vi "Main.vi"() -> ()   [LabVIEW 2019]
doc: "The myRIO Project template acquires acceleration data from the onboard accelerometer and displays the changes of acceleration values in a waveform chart."
uses:
  <vilib>/myRIO/Common/Instrument Driver Framework/myRIO v1.0/Encoder/typedefs/Encoder Signal Mode.ctl
  <vilib>/myRIO/Instrument Drivers/Onboard IO/Encoder/typedefs/Encoder Reference.ctl
  <vilib>/myRIO/Common/Instrument Driver Framework/Utilities/typedefs/myRIO Generic Hardware Reference.ctl
  <vilib>/myRIO/Common/Instrument Driver Framework/Utilities/typedefs/Hardware Version Enum.ctl
  <vilib>/myRIO/Common/Instrument Driver Framework/Utilities/typedefs/myRIO v1.0 Reference.ctl
  <vilib>/myRIO/Common/Instrument Driver Framework/Utilities/typedefs/Generic FPGA Reference.ctl
  <vilib>/myRIO/Common/Instrument Driver Framework/myRIO v1.0/Encoder/typedefs/Encoder Channels Enum.ctl
  <vilib>/myRIO/Common/Instrument Driver Framework/myRIO v1.0/Encoder/typedefs/Encoder Configuration v1.0.ctl
  <vilib>/userDefined/High Color/nirio_resource_hc.ctl
  <vilib>/Simulation/Scripting/Companion Diagram/SimConfigNode/SimParams.ctl
  <vilib>/Simulation/Scripting/Companion Diagram/SimConfigNode/_simSolvers.ctl
  <vilib>/Simulation/Implementation/Shared/SIMSCR Execution Mode.ctl
  <vilib>/Simulation/Param Hierarchy/Typedefs/SIMPH Param Control Actions.ctl
  <vilib>/myRIO/Common/Instrument Driver Framework/Utilities/vis/Is FPGA Ref Available.vi
  <vilib>/myRIO/Common/Instrument Driver Framework/myRIO v1.0/Encoder/vis/myRIO v1.1 Open Encoder.vi
  <vilib>/myRIO/Instrument Drivers/Onboard IO/Encoder/vis/Read.vi
  <vilib>/Simulation/Implementation/Shared/NILVSim_ParamChanged.vi
  <vilib>/Simulation/Implementation/Shared/NILVSIM_BeginStep.vi
  <vilib>/Simulation/Implementation/Shared/NILVSim_Manager.vi
  <vilib>/Utility/error.llb/Clear Errors.vi
  <vilib>/Simulation/Implementation/Shared/NILVSim_FinalizeModel.vi
  <vilib>/myRIO/Common/Instrument Driver Framework/Utilities/vis/Validate Channels.vi
  <vilib>/myRIO/Common/Instrument Driver Framework/myRIO v1.0/Encoder/vis/myRIO v1.0 Reserve Encoder.vi
  <vilib>/myRIO/Common/Instrument Driver Framework/myRIO v1.0/UART/vis/myRIO v1.0 Close UART.vi
  <vilib>/myRIO/Common/Instrument Driver Framework/myRIO v1.0/Encoder/vis/myRIO v1.0 Build MUX Configuration Encoder.vi
  <vilib>/myRIO/Common/Instrument Driver Framework/myRIO v1.0/Resource Manager/vis/myRIO v1.0 Reserve Channel List.vi
  <vilib>/myRIO/Common/Instrument Driver Framework/myRIO v1.0/Resource Manager/vis/myRIO v1.0 Create Configuration List.vi
  <vilib>/myRIO/Common/Instrument Driver Framework/myRIO v1.0/Resource Manager/vis/myRIO v1.0 Reserve Channel.vi
  <vilib>/myRIO/Common/Instrument Driver Framework/myRIO v1.0/Resource Manager/vis/myRIO v1.0 Unreserve Channel.vi
  <vilib>/myRIO/Common/Instrument Driver Framework/myRIO v1.0/Resource Manager/vis/myRIO v1.0 Build Mutex Name.vi
  <vilib>/Utility/VariantDataType/GetNumericInfo.vi
  <vilib>/Utility/error.llb/Error Cluster From Error Code.vi
  <vilib>/myRIO/Common/Instrument Driver Framework/myRIO v1.0/myRIO v1.1 Open.vi
  <vilib>/myRIO/Common/Instrument Driver Framework/Utilities/vis/IO Manager.vi
  <vilib>/myRIO/Common/Instrument Driver Framework/Utilities/vis/Configuration Manager.vi
  <vilib>/myRIO/Common/Instrument Driver Framework/myRIO v1.0/Resource Manager/vis/myRIO v1.0 Configure IO.vi
  <vilib>/myRIO/Common/Instrument Driver Framework/myRIO v1.0/myRIO v1.0 Close.vi
  <vilib>/myRIO/Common/Instrument Driver Framework/myRIO v1.0/Encoder/vis/myRIO v1.0 Configure Encoder.vi
  <vilib>/myRIO/Common/Instrument Driver Framework/myRIO v1.0/Encoder/vis/myRIO v1.0 Read Encoder.vi
  <vilib>/Simulation/Implementation/Shared/SIM Unbundle Sim Info.vi
  <vilib>/Simulation/Implementation/Shared/NILVSim_Initialize.vi
  <vilib>/Simulation/Utility/Implementation/NILVSim Get Time and IsAcceptedStep.vi
  <vilib>/Simulation/Implementation/Shared/SIMSH Read Queue.vi
  <vilib>/Simulation/Implementation/Shared/NILVSim_GetModelError.vi
  <vilib>/Simulation/Implementation/Shared/SIM Bundle Sim Info.vi
  <vilib>/Utility/file.llb/Write Delimited Spreadsheet (DBL).vi
  <vilib>/myRIO/Common/Instrument Driver Framework/Utilities/vis/FPGA Ref Manager.vi
  <vilib>/myRIO/Common/Instrument Driver Framework/myRIO v1.0/myRIO v1.0 Reset FPGA.vi
  <vilib>/myRIO/Common/Instrument Driver Framework/myRIO v1.0/IRQ/vis/myRIO v1.0 IRQ Info FGV.vi
  <vilib>/myRIO/Common/Instrument Driver Framework/myRIO v1.0/IRQ/vis/myRIO v1.0 Timer IRQ Info FGV.vi
  <vilib>/myRIO/Common/Instrument Driver Framework/myRIO v1.0/IRQ/vis/myRIO v1.0 ISR Agent.vi
  <vilib>/myRIO/Instrument Drivers/Utilities/vis/Reset Index.vi
  <vilib>/myRIO/Common/Instrument Driver Framework/myRIO v1.0/Resource Manager/vis/myRIO v1.0 Block Write Resource Manager.vi
  <vilib>/myRIO/Express VI/Onboard IO/Encoder/Encoder Express VI.xnode
  <vilib>/myRIO/Common/Instrument Driver Framework/myRIO v1.0/Encoder/typedefs/Encoder Count Direction Enum.ctl
  <vilib>/myRIO/Instrument Drivers/Onboard IO/Encoder/vis/myRIO Encoder Open.xnode
  <vilib>/Simulation/Implementation/XNodeFramework/SimXNode/SimX.xnode
  Sub_OBS.vi
  <vilib>/Simulation/Scripting/Companion Diagram/SimConfigNode/SimDog.xnode
  <vilib>/myRIO/Instrument Drivers/Onboard IO/Encoder/Encoder.lvlib
  <vilib>/myRIO/Instrument Drivers/Utilities/Utilities.lvlib
  <vilib>/Simulation/Implementation/Shared/NI_SIM_Implementation.lvlib
panel:
  out "error out":errorcluster
  in  "Stop 2":bool
  out "Direction 1":enum16{"Counting Up", "Counting Down"}(ring)
  out "Overflow? 1":bool
  in  "Reset":bool
  out "Graph 3":T1(graph)
  in  "Freq[Hz]":dbl=1000.0
  out "Direction 2":enum16{"Counting Up", "Counting Down"}(ring)
  out "Overflow? 2":bool
  in  "Reset 2":bool
  out "ref pos 2":dbl
  out "Duty Cycle out 2":dbl=0.5
  out "Duty Cycle out":dbl=0.5
  in  "k_OBS":dbl
  in  "b_OBS":dbl=1.0
  in  "b_TAR":dbl
  in  "k_TAR":dbl=1.0
  out "Graph 2":cluster{dbl, "x2hat":dbl}(graph)
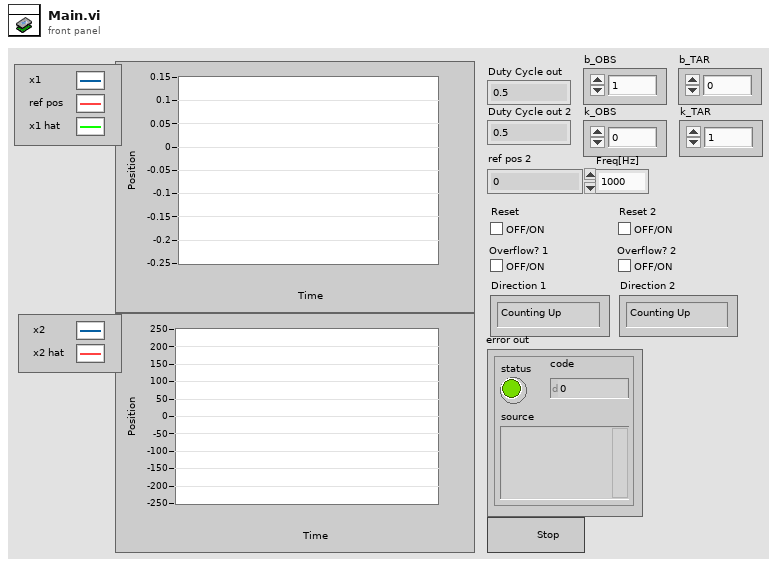
[diagram p1: front panel]
types:
  T1 = cluster{"ave out":dbl, "ave out":dbl, "x1hat":dbl}
  T2 = enum16{"Simulate to Completion", "Single Time-Step Simulation (Fixed Step Only)"}
  T3 = typedef "SIMSCR Execution Mode.ctl" = enum16{"Simulate to Completion", "Single Time-Step Simulation (Fixed Step Only)"}
  T4 = typedef "SIMPH Param Control Actions.ctl" = enum16{"get params", "set params"}
  T5 = cluster{"SIMSH Sim Time":dbl, "Sum 3":cluster{"Result":dbl}, "L2":cluster{"output":dbl}, "L1":cluster{"output":dbl}, "Summation 2":cluster{"Result":dbl}, "Formula Node":cluster{"AI":dbl, "BI":dbl, "L1":dbl, "L2":dbl}, "A/I":cluster{"output":dbl}, "2":cluster{"output":dbl}, "1":cluster{"output":dbl}, "Summation":cluster{"Result":dbl}, "B/I":cluster{"output":dbl}}
  T6 = typedef "SimParams.ctl" = cluster{"Initial Time (s)":dbl, "Final Time (s)":dbl, "Step Size (s)":dbl, "ODE Solver":T7, "Minimum Step Size (s)":dbl, "Maximum Step Size (s)":dbl, "Relative Tolerance":dbl, "Absolute Tolerance":dbl, "Software Timing":bool, "Initial Step Size (s)":dbl, "Automatic Fixed Step Size?":bool, "Automatic Discrete Step Size?":bool, "Discrete Step Size (s)":dbl, "Calculate using Time Step":bool, "Solver Wired?":bool, "Prev.Frm.Expected End":u64, "Prev.Frm.Actual End":u64, "Prev.Frm.Finished Late?":bool, "Prev.Iter.Expected End":u64, "Prev.Iter.Actual End":u64, "Prev.Iter.Finished Late?":bool, "Expected Iteration Start":u64, "Actual Iteration Start":u64, "Expected Frame Start":u64, "Actual Frame Start":u64, "Source Name":string, "Name":string, "Period":i64, "Deadline":i64, "Offset":i64, "Start":i64, "Priority":i32, "Timeout":i32, "Processor":i32, "Mode":enum32{"No Change", "Process missed periods, maintain original phase", "Discard missed periods, maintain original phase", "Process missed periods, ignore original phase", "Discard missed periods, ignore original phase"}, "Wakeup reason":enum32{"Normal", "Aborted", "Asynchronous wakeup", "Timing source error", "Timed loop error", "Timeout"}, "Error":errorcluster, "Source Type":string, "Secondary Source Type":string, "Global End Time":u64, "Global Start Time":u64, "Full Solver Reset":bool, "Execution Mode":T3, "Nan/Inf Check":bool, "Custom Solver Library":string, "Solver Is Variable":bool, "custom solver name":string, "Signal Collection Decimation":u32}
  T7 = typedef "_simSolvers.ctl" = enum16{"Runge-Kutta 1 (Euler)", "Runge-Kutta 2", "Runge-Kutta 3", "Runge-Kutta 4", "Runge-Kutta 23 (variable)", "Runge-Kutta 45 (variable)", "BDF (variable)", "Adams-Moulton (variable)", "Rosenbrock (variable)", "Discrete States Only", "SDIRK 4 (variable)", "Radau 5 (variable)", "Radau 9 (variable)", "Radau 13 (variable)", "Radau [Variable Order] (variable)", "Gear's Method (variable)", "Linearizer", "State Query", "Trim Eval", "Custom Solver"}
  T8 = typedef "Encoder.lvlib/Encoder Reference.ctl" = cluster{"myRIO Reference":T9, "Encoder Channels Enum":T13}
  T9 = typedef "myRIO Generic Hardware Reference.ctl" = cluster{"myRIO Model":T10, "myRIO Hardware Reference":T11}
  T10 = typedef "Hardware Version Enum.ctl" = enum16{"Unknown", "myRIO-1900", "myRIO-1950", "roboRIO", "NI ELVIS RIO CM", "ELVIS III"}
  T11 = typedef "myRIO v1.0 Reference.ctl" = cluster{"Generic FPGA Reference":T12, "Allow multiple opens":bool}
  T12 = typedef "Generic FPGA Reference.ctl" = refnum<k20>
  T13 = typedef "Encoder Channels Enum.ctl" = enum16{"Not Connected", "C/ENC0", "C/ENC1", "A/ENC", "A/ENC0", "A/ENC1", "A/ENC2", "A/ENC3", "A/ENC4", "A/ENC5", "A/ENC6", "A/ENC7", "A/ENC8", "A/ENC9", "B/ENC", "B/ENC0", "B/ENC1", "B/ENC2", "B/ENC3", "B/ENC4", "B/ENC5", "B/ENC6", "B/ENC7", "B/ENC8", "B/ENC9", "DIO/ENC0", "DIO/ENC1", "DIO/ENC2", "DIO/ENC3", "DIO/ENC4"}
  T14 = typedef "Encoder Signal Mode.ctl" = enum16{"Quadrature phase signal", "Step and direction signal"}
  T15 = typedef "nirio_resource_hc.ctl" = tag
  T16 = typedef "Encoder Count Direction Enum.ctl" = enum16{"Counting Up", "Counting Down"}
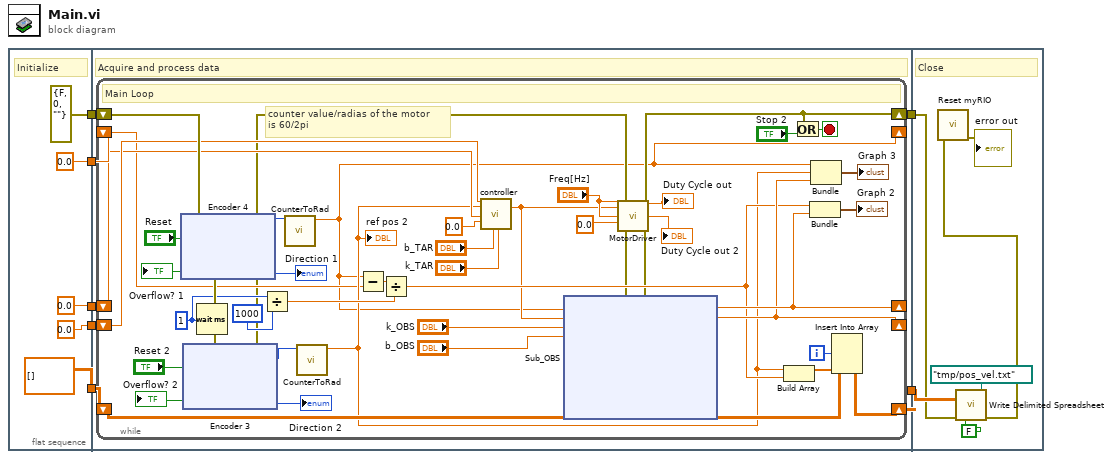
[diagram p0: block diagram]
diagram:
  n1 = flat-sequence {
    tunnel: [errorcluster {"status"=FALSE, "code"=0, "source"=""} ("error in (no error)")] -> w7
    tunnel: [dbl[][] [] ("array")] -> w6
    tunnel: [0.0 ("rads")] -> w5
    tunnel: [0.0 ("rads")] -> w4
    tunnel: [0.0 ("rads")] -> w3
    tunnel: w7 -> [w19]
    tunnel: w6 -> [w18]
    tunnel: [w17] -> w2
    tunnel: [w16] -> w1
    tunnel: w5 -> [w15]
    tunnel: w4 -> [w14]
    tunnel: w3 -> [w13]
    tunnel: w2 -> [w430]
    tunnel: w1 -> [w431]
    frame #0 {
      # "Initialize"
    }
    frame #1 {
      # "Acquire and process data"
      n2 = while {
        shift-right: [w47] -> w17
        shift-left: w19 -> [w53]
        shift-right: [w56] -> w16
        shift-left: w18 -> [w55]
        shift-right: [w20] -> _
        shift-left: w15 -> [w24]
        shift-right: [w30] -> _
        shift-left: w13 -> [w29]
        shift-right: [w31] -> _
        shift-left: w14 -> [w28]
        i -> [w52]
        stop <- w61 stop-if-true
        w41 = u32 1 ("milliseconds to wait")
        # "counter value/radias of the motor \nis 60/2pi"
        # "Main Loop"
        n3 = xnode "Encoder 4"("error in (no error)"=w53, "Reset Counter"="Reset") -> ("error out"=w46:errorcluster, "Counter Value"=w57:i32, "Counter Direction"=→"Direction 1":T16, "Overflow?"=→"Overflow? 1":bool)
        n4 = xnode "Encoder 3"("error in (no error)"=w46, "Reset Counter"="Reset 2") -> ("error out"=w21:errorcluster, "Counter Value"=w48:i32, "Counter Direction"=→"Direction 2":T16, "Overflow?"=→"Overflow? 2":bool)
        n5 = Wait (ms)(milliseconds to wait=w41) -> ()  [unwired: 1 out]
        n6 = Divide(x=w41, y=u32 1000) -> (x/y=w44:dbl)
        n7 = call "CounterToRad.vi"("Counter Value"=w57) -> ("rads"=w20:dbl)  [unwired: 10 in]
        n8 = call "CounterToRad.vi"("Counter Value"=w48) -> ("rads"=w25:dbl)  [unwired: 10 in]
        "ref pos 2" <- w25
        n9 = Subtract(x=w20, y=w24) -> (x-y=w43:dbl)
        n10 = Divide(x=w43, y=w44) -> (x/y=w26:dbl)
        n11 = call "controller.vi"("position"=w29, "pos ref"=w25, "velocity"=w28, "vel ref"=0.0, "K2"="b_TAR", "K1"="k_TAR") -> ("duty out"=w23:dbl)  [unwired: 13 in]
        n12 = xnode "Sub_OBS"("Yin"=w20, "DutyCycle_OBS"=w23, "k_OBS"="k_OBS", "b_OBS"="b_OBS", "error in"=w21) -> ("x2hat"=w31:dbl, "x1hat"=w30:dbl, "error out"=w22:errorcluster)  [unwired: 1 in, 6 out]
        n13 = call "MotorDriver.vi"("Frequency [Hz]"="Freq[Hz]", "Duty Cycle in"=w23, "Frequency [Hz] 2"="Freq[Hz]", "Duty Cycle in 2"=0.0, "error in (no error)"=w22) -> ("Duty Cycle out"=→"Duty Cycle out":dbl, "Duty Cycle out 2"=→"Duty Cycle out 2":dbl, "error out"=w47:errorcluster)  [unwired: 8 in]
        n14 = Build Array(w25, w26) -> (w54:dbl[])
        n15 = Or(x=w47, y="Stop 2") -> (x .or. y?=w61:bool)
        n16 = Bundle(w26, "x2hat"=w31) -> (→"Graph 2":cluster{dbl, "x2hat":dbl})  [unwired: 1 in]
        n17 = Bundle("rads"=w20, "rads"=w25, "x1hat"=w30) -> (→"Graph 3":cluster{"rads":dbl, "rads":dbl, "x1hat":dbl})  [unwired: 1 in]
        n18 = Insert Into Array(array=w55, index (row)=w52, new element=w54) -> (w56:dbl[][])  [unwired: 1 in]
      }
    }
    frame #2 {
      # "Close"
      n19 = call-poly <vilib>:"Write Delimited Spreadsheet.vi"("file path (dialog if empty)"=path "/tmp/pos_vel.txt", "2D data"=w431, "error in (no error)"=w430, "transpose? (no:F)"=FALSE) -> ("error out"=w429:errorcluster)  [unwired: 10 in, 1 out]
      n20 = call <vilib>:"Reset myRIO.vi"("error in (no error)"=w429) -> ("error out"=→"error out":errorcluster)  [unwired: 10 in]
    }
  }
